vi "Trip Log and Trip Monitor.vi"(8 "error in (no error)":errorcluster, 11 "main ref":T1) -> (0 "error out":errorcluster)   [LabVIEW 2025]
uses:
  v06/controls/LAB-IQ UI Data.ctl
  Traction Loop/Traction Receipe Enum.ctl
  HEAVE vi's/Heave Write enum.ctl
  <vilib>/Utility/error.llb/Trim Whitespace One-Sided.vi
  Temperature/Temperature enum.ctl
panel:
  out "error out 4":errorcluster
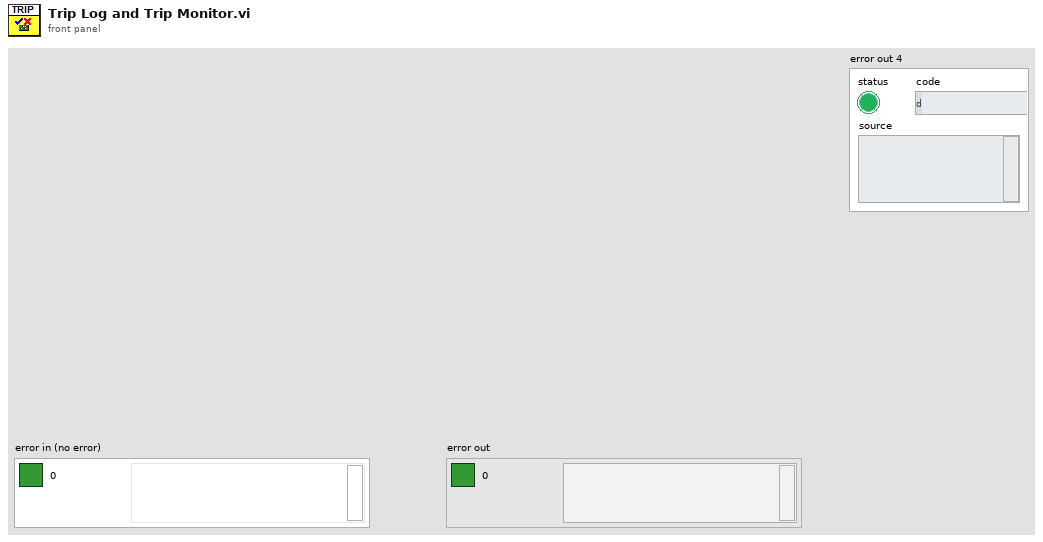
[diagram p1: front panel]
types:
  T1 = typedef "LAB-IQ UI Data.ctl" = cluster{"Main Home Screen":cluster{"GUI":refnum<vi>, "Platform Settings":refnum<vi>, "Configure":refnum<vi>, "Home":refnum<vi>, "EXIT":refnum<vi>, "service 2":refnum<vi>, "MainPage":refnum<vi>, "Analysis":refnum<vi>}, "Platform Settings":cluster{"mm/s  Surge":refnum<vi>, "Drive Error":refnum<vi>, "Disable Axis Jog Soft Limits":refnum<vi>, "mm/s  Sway":refnum<vi>, "Sway and Surge COM Status":refnum<vi>, "Heave COM Status":refnum<vi>, "Enable Platform":refnum<vi>, "Surge Forward Main":refnum<vi>, "Sway Right Main":refnum<vi>, "Sway Left Main":refnum<vi>, "Heave Down Main":refnum<vi>, "Heave Up main":refnum<vi>, "mm/s Heave":refnum<vi>, "mm/sec":refnum<vi>, "mm":refnum<vi>, "Surge Backward Main":refnum<vi>}, "Analysis Screen":cluster{"Analysis Home":refnum<vi>, "Surface Analysis":refnum<vi>, "Imaging":refnum<vi>, "Image Analysis":refnum<vi>, "Post Analysis":refnum<vi>}, "Config Screen":cluster{"Select Load Head":refnum<vi>, "Notes :":refnum<vi>, "FILE":refnum<vi>, "Sample ID :":refnum<vi>, "Operator ID :":refnum<vi>, "Operator Name :":refnum<vi>, "Auto":refnum<vi>}, "Motion Module":cluster{"zNL":refnum<vi>, "NL disp":refnum<vi>, "Rotary Tab":refnum<vi>, "Motion Direction:  3":refnum<vi>, "E.Velocity 2":refnum<vi>, "e.v/ssr 2":refnum<vi>, "Enter Fixed E.Velocity 2":refnum<vi>, "Enter Final SRR 2":refnum<vi>, "Enter initial SRR 2":refnum<vi>, "Enter Fixed SRR 2":refnum<vi>, "Enter the Final E.Velocity (m/s) 2":refnum<vi>, "Enter initial E.Velocity (m/s) 2":refnum<vi>, "Final Speed (RPM) 3":refnum<vi>, "Initial Speed (RPM) 2":refnum<vi>, "Enter the Final Velocity (m/s) 3":refnum<vi>, "Enter initial Velocity (m/s)  3":refnum<vi>, "Ramp Up 2":refnum<vi>, "TEST SELECTION":refnum<vi>, "SPEED SELECTION : ":refnum<vi>, "Angular Oscillation Set":refnum<vi>, "Traction":refnum<vi>, "Step Speed":refnum<vi>, "StepTable For Load-Speed":refnum<vi>, "StepTable For Speed":refnum<vi>, "Surge Forward MM":refnum<vi>, "Surge Backward MM":refnum<vi>, "M3 Image":refnum<vi>, "String 39":refnum<vi>, "Sway Left MM":refnum<vi>, "Sway Right MM":refnum<vi>, "Disable Axis Jog Soft Limits":refnum<vi>, "mm":refnum<vi>, "Heave Down MM":refnum<vi>, "Heave Up MM":refnum<vi>, "Wear Track Diameter (mm)":refnum<vi>, "Set WTD":refnum<vi>, "HomeScratch":refnum<vi>, "HomeRot":refnum<vi>, "PlaceModule":refnum<vi>, "Enter the Angle (Deg)":refnum<vi>, "Enter the Frequency (Hz)":refnum<vi>, "Motion Mode:":refnum<vi>, "LR Sway":refnum<vi>, "Rot Hor":refnum<vi>, "Scratch":refnum<vi>, "LR Cam":refnum<vi>, "MMBack":refnum<vi>, "MMNext":refnum<vi>, "Rot Ver":refnum<vi>, "Rotary Module Selection":refnum<vi>, "calculate rotary":refnum<vi>, "SPEED SELECTION : rotary":refnum<vi>, "Import 2":refnum<vi>, "Save 2":refnum<vi>, "File Path :  2":refnum<vi>, "String 45":refnum<vi>, "StepTable For Speed 3":refnum<vi>, "Enter the Speed(mm/sec)":refnum<vi>, "Enter the Speed(RPM)":refnum<vi>, "Enter Scratch Speed (mm/s):":refnum<vi>, "SwaySpeed Set":refnum<vi>, "Scartch Offset":refnum<vi>, "Motion type:":refnum<vi>, "HomeScratch 2":refnum<vi>, "Enter Scratch length (mm):":refnum<vi>, "Wear Track Diameter":refnum<vi>, "Rotary Speed Exced":refnum<vi>, "Scratch Mode":refnum<vi>, "No of Scratch":refnum<vi>}, "Environmental control":cluster{"Humidity  Status  3":refnum<vi>, "Low Temp  Status  2":refnum<vi>, "TK4 status 2":refnum<vi>, "Stage Temperature":refnum<vi>, "Sample Temperature":refnum<vi>, "Humidity (Amb)":refnum<vi>, "Clear List":refnum<vi>, "Add to list":refnum<vi>, "Wear":refnum<vi>, "Vibration":refnum<vi>, "Humidity (Chamber)":refnum<vi>, "Temperature (Chamber)":refnum<vi>, "ECR ":refnum<vi>, "Temperature (Amb)":refnum<vi>, "Microphone":refnum<vi>, "Acoustic Emission 3":refnum<vi>, "SNext":refnum<vi>, "APBack":refnum<vi>, "Enter the Temperature (°C):":refnum<vi>, "Enter the Stage \nTemperature (°C):":refnum<vi>, "Enter the Humidity (%Rh):":refnum<vi>, "Low Temp":refnum<vi>, "High Temp":refnum<vi>, "Humidity":refnum<vi>, "Sensors Picked":refnum<vi>}, "About Screen":cluster{"Password":refnum<vi>, "Home Service":refnum<vi>, "Advanced Setting":refnum<vi>, "About Tab":refnum<vi>, "ECR Port:":refnum<vi>, "Ramp Port:":refnum<vi>, "Installation/Replacement completed":refnum<vi>, "Loahead":refnum<vi>, "Heave and Surge COM Port:":refnum<vi>, "Sway COM Port:":refnum<vi>, "Temp Modbus:":refnum<vi>, "Humidity Port:":refnum<vi>, "Edit Gain Constants":refnum<vi>, "Save Gain Constants":refnum<vi>}, "Main Screen":cluster{"Main Screen Tab":refnum<vi>, "Angle and Frequency":refnum<vi>, "Stroke (mm)":refnum<vi>, "Angle (Deg)":refnum<vi>, "Main Speed Tab":refnum<vi>, "MTM MOTOR DISPLAY":refnum<vi>, "Disc Speed (m/sec)":refnum<vi>, "Ball Speed (m/sec)":refnum<vi>, "Disc Speed (RPM)":refnum<vi>, "Ball Speed (RPM)":refnum<vi>, "SPEED TAB":refnum<vi>, "Speed (m/sec)":refnum<vi>, "Set Speed (m/sec)":refnum<vi>, "Speed (RPM)":refnum<vi>, "Set Speed":refnum<vi>, "Time Tab":refnum<vi>, "Time ( HH:MM:SS ) 2":refnum<vi>, "Test Duration":refnum<vi>, "Test Duration 4":refnum<vi>, "TEST CYCLE":refnum<vi>, "TOTAL CYCLES":refnum<vi>, "Set Load (N)":refnum<vi>, "Temp Tabs":refnum<vi>, "Heater":refnum<vi>, "TK4 status":refnum<vi>, "ChamberTemp":refnum<vi>, "SetTmp":refnum<vi>, "Controller  Status":refnum<vi>, "ChamberTemp 2":refnum<vi>, "SetTmp 2":refnum<vi>, "Controller  Status 2":refnum<vi>, "ChamberTemp 3":refnum<vi>, "SetTmp 3":refnum<vi>, "Cooling":refnum<vi>, "Load Communication":refnum<vi>, "Ambient \nTemperature":refnum<vi>, "HumCOMStatus":refnum<vi>, "Ambient\n Humidity":refnum<vi>, "Freq (Hz)":refnum<vi>, "Load En":refnum<vi>, "NLt":refnum<vi>, "zNL 2":refnum<vi>, "Humidity On":refnum<vi>, "humidity disp":refnum<vi>, "Set Humidity":refnum<vi>, "NL disp 2":refnum<vi>, "Humidity On 2":refnum<vi>, "humidity disp 2":refnum<vi>, "Set Humidity 2":refnum<vi>, "NL disp 3":refnum<vi>, "AppLoadSeq scratch":refnum<vi>, "Stop Scratch":refnum<vi>, "ClrLog":refnum<vi>, "Trip Log":refnum<vi>, "STOP":refnum<vi>, "Start Test":refnum<vi>, "Test status":refnum<vi>, "AR Led":refnum<vi>, "Data":refnum<vi>, "Health":refnum<vi>, "Sway COM Status":refnum<vi>, "Heave COM Status":refnum<vi>, "Grp Tab":refnum<vi>, "Sub Graph":refnum<vi>, "SD (mm)":refnum<vi>, "Siliding distance Reset Graph":refnum<vi>, "SDGp":refnum<vi>, "Humidity Reset Graph":refnum<vi>, "HumrGp":refnum<vi>, "Acoustic Emission (mV)":refnum<vi>, "Aqucostic Reset Graph":refnum<vi>, "gACQUOS":refnum<vi>, "ECR RESET":refnum<vi>, "ECR":refnum<vi>, "Temperature Reset":refnum<vi>, "Acoustic Emission (mV) 2":refnum<vi>, "Aqucostic Reset Graph 2":refnum<vi>, "gACQUOS 2":refnum<vi>, "ECR RESET 2":refnum<vi>, "ECR 2":refnum<vi>, "Temperature Reset 2":refnum<vi>, "Temperature (deg c)":refnum<vi>, "Speed Reset Graph":refnum<vi>, "Speed Tab":refnum<vi>, "MTM DISC  SPEED":refnum<vi>, "MTM BALL SPEED":refnum<vi>, "speed mm/sec":refnum<vi>, "Hymidity":refnum<vi>, "Humidity Disable trip":refnum<vi>, "CoF Trip  2":refnum<vi>, "Depth Trip":refnum<vi>, "Weart Deapth":refnum<vi>, "Depth Reset Graph":refnum<vi>, "Weart":refnum<vi>, "Depthz":refnum<vi>, "Depth (µm)":refnum<vi>, "WearGp":refnum<vi>, "NL Trip 2":refnum<vi>, "Load pid":refnum<vi>, "Load Disable Trip":refnum<vi>, "Load Reset Graph":refnum<vi>, "NL Display 4":refnum<vi>, "Main Chart 3":refnum<vi>, "BACK":refnum<vi>, "Depth Trip 2":refnum<vi>, "COF TRIP ":refnum<vi>, "Friction Force (N)":refnum<vi>, "FF Reset Graph":refnum<vi>, "FF Disable Trip":refnum<vi>, "FF TRIP":refnum<vi>, "COF Disable Trip":refnum<vi>, "COF Reset Graph":refnum<vi>, "Start Test Temp":refnum<vi>, "zFF":refnum<vi>, "Friction Force (N) Graph":refnum<vi>, "Coefficient of Friction":refnum<vi>, "Scratch Start Test":refnum<vi>, "FF Tab":refnum<vi>, "Cyclic Friction Force (N)":refnum<vi>, "CZ FF":refnum<vi>, "Cyclic Friction Force (N) Graph":refnum<vi>, "Cyclic Coefficient of Friction":refnum<vi>, "Cyclic FF TRIP":refnum<vi>, "Cyclic FF Disable Trip":refnum<vi>, "cyclic COF Disable Trip":refnum<vi>, "cyclic COF TRIP":refnum<vi>, "cyclic COF Reset Graph":refnum<vi>, "Cyclic FF Reset Graph":refnum<vi>, "Test Trip":refnum<vi>, "Multi Scratch Pass":refnum<vi>, "Scratch Start Recording":refnum<vi>, "Coefficient of Friction 2":refnum<vi>, "Acoustic Emission":refnum<vi>, "Friction Force (N) 2":refnum<vi>, "Depth (Microns)":refnum<vi>, "Normal Load ( N )":refnum<vi>}, "Loading":cluster{"Indentation":refnum<vi>, "Reference Sample":refnum<vi>, "Load Cell Communication Slide":refnum<vi>, "com 3":refnum<vi>, "com":refnum<vi>, "DecaForce COM Status":refnum<vi>, "Update":refnum<vi>, "Clear 3":refnum<vi>, "seq":refnum<vi>, "Stribeck table":refnum<vi>, "Stribeck Table  For loading":refnum<vi>, "Loading Mode":refnum<vi>, "Enter the Final Load (N)":refnum<vi>, "Enter the CoF Trip":refnum<vi>, "Enter the Friction Force Trip":refnum<vi>, "Enter the Normal load Trip":refnum<vi>, "Enter the Load  (N)":refnum<vi>, "KiloForce":refnum<vi>, "DecaForce ":refnum<vi>, "MicroForce":refnum<vi>, "LHBack":refnum<vi>, "LHNext":refnum<vi>, "Enter the Loading Rate (N/min)":refnum<vi>, "Message":refnum<vi>, "Warning 2":refnum<vi>, "SSP 0.75":refnum<vi>, "SSP 0.5":refnum<vi>, "SSP 0.3":refnum<vi>, "Warning":refnum<vi>, "gui GIF":refnum<vi>, "Communication is established":refnum<vi>, "AppLoad 4":refnum<vi>, "Multipoint":refnum<vi>, "Load Selection":refnum<vi>}, "PID":cluster{"Ramp":refnum<vi>, "Vertical load (N)":refnum<vi>, "apply load":refnum<vi>, "apply load 2":refnum<vi>, "Enter ByPass Load":refnum<vi>, "Bypass Load":refnum<vi>, "gFF Rot":refnum<vi>}, "Config Parameters":cluster{"Tab Control 3":refnum<vi>, "Tab Control 19":refnum<vi>, "SAMPLES":refnum<vi>, "Re-initilaize":refnum<vi>, "Filter ON/OFF":refnum<vi>, "TracHomeSurgeOffsetCounts 10MM":refnum<vi>, "TracHomeSwayOffsetCounts 10MM":refnum<vi>, "Acoustic Emission:":refnum<vi>, "Apply Filter (FF)":refnum<vi>, "Filter% 2":refnum<vi>, "Apply Filter (Load)":refnum<vi>, "Filter% ":refnum<vi>, "Sway distance (mm)":refnum<vi>, "Surge distance (mm)":refnum<vi>, "DataSavingLoopDelay(ms)":refnum<vi>, "SAVE 2":refnum<vi>, "Enter Distance":refnum<vi>, "Sway Counts:":refnum<vi>, "Distance (mm): 3":refnum<vi>, "Surge Counts:":refnum<vi>, "Distance (mm): 2":refnum<vi>, "Distance (mm):":refnum<vi>, "Heave Counts:":refnum<vi>, "LRMHomeSurgeOffsetCounts":refnum<vi>, "LRMHomeSwayOffsetCounts":refnum<vi>, "TracHomeSurgeOffsetCounts 20MM":refnum<vi>, "TracHomeSwayOffsetCounts 20MM":refnum<vi>, "RotHomeSwayOffsetCounts":refnum<vi>, "RotHomeSurgeOffsetCounts":refnum<vi>, "Heave distance":refnum<vi>, "Zmm":refnum<vi>, "Heave Pulses/mm":refnum<vi>, "Surge Pulses/mm":refnum<vi>, "Sway Pulses/mm":refnum<vi>, "Heave Pitch":refnum<vi>, "Surge Pitch":refnum<vi>, "Sway Pitch":refnum<vi>, "Heave PPR":refnum<vi>, "Surge PPR":refnum<vi>, "Sway PPR":refnum<vi>, "Tab Control 5":refnum<vi>, "Tab Control 14":refnum<vi>, "Tab Control 26":refnum<vi>, "AE":refnum<vi>, "Heave Loop Delay":refnum<vi>, "Heave PID Speed":refnum<vi>, "Surge Jog Speed":refnum<vi>, "Heave Jog Speed":refnum<vi>, "Sway Loop Delay":refnum<vi>, "Sway PID Speed":refnum<vi>, "Sway Jog Speed":refnum<vi>, "DEPTH TRIP VALUE":refnum<vi>, "LOAD TRIP VALUE":refnum<vi>, "DEPTH TRIP   ENABLE":refnum<vi>, "LOAD TRIP  ENABLE":refnum<vi>, "CYCLIC FF TRIP VALUE":refnum<vi>, "FF TRIP VALUE":refnum<vi>, "CYCLIC CoF TRIP VALUE":refnum<vi>, "COF TRIP VALUE":refnum<vi>, "CYCLIC COF TRIP  ENABLE":refnum<vi>, "CYCLIC FF TRIP  ENABLE":refnum<vi>, "FF TRIP  ENABLE":refnum<vi>, "COF TRIP  ENABLE":refnum<vi>, "JOG TRIP LOAD VALUE (N)":refnum<vi>, "Rotary Vertical":refnum<vi>, "Traction":refnum<vi>, "Scratch":refnum<vi>, "LRM CAM":refnum<vi>, "Sway LRM":refnum<vi>, "Rotary Horizontal":refnum<vi>, "SURGE SPEED":refnum<vi>, "SURGE BACKWARD COUNT":refnum<vi>, "SURGE FORWARD COUNT":refnum<vi>, "Start Button":refnum<vi>}, "Loading Com Port":cluster{"ClearAll":refnum<vi>, "Mz(Nm)":refnum<vi>, "My(Nm)":refnum<vi>, "Mx(Nm)":refnum<vi>, "Save Dwell":refnum<vi>, "Acq Delay (ms)":refnum<vi>, "Burst Delay (ms)":refnum<vi>, "model":refnum<vi>, "SN":refnum<vi>, "FFx(N)":refnum<vi>, "Sensor IP":refnum<vi>, "Port":refnum<vi>, "FFy(N)":refnum<vi>, "Load(N)":refnum<vi>, "delete Handle":refnum<vi>, "Create Handle":refnum<vi>, "ft_data":refnum<vi>, "ft_range":refnum<vi>, "ft_data 2":refnum<vi>, "stop 6":refnum<vi>, "running_flag":refnum<vi>, "ft_udp_handle":refnum<vi>, "get-data-return":refnum<vi>, "get-range-return":refnum<vi>, "zero-return":refnum<vi>, "filter-return":refnum<vi>, "initial-return":refnum<vi>, "deleteHandle-result":refnum<vi>, "Load Cell Temp":refnum<vi>, "Load Cell":refnum<vi>, "ZeroAll":refnum<vi>, "FORCE (N)":refnum<vi>, "TORQUE (N-m)":refnum<vi>, "Load Cell Link":refnum<vi>}, "Heave AND Surge":cluster{"SURGE POSE":refnum<vi>, "error out Read":refnum<vi>, "HEAVE POSE":refnum<vi>, "State":refnum<vi>, "Homed":refnum<vi>, "Sequence ID":refnum<vi>, "error out Write":refnum<vi>, "faultCode":refnum<vi>, "Ack ID":refnum<vi>, "SPEED":refnum<vi>, "Distance":refnum<vi>, "Mode Command":refnum<vi>, "Heave and Surge Read":refnum<vi>, "Read Heave Temp":refnum<vi>, "Spare 15":refnum<vi>, "Spare 14":refnum<vi>, "Spare 13":refnum<vi>, "Spare 12":refnum<vi>, "Spare 11":refnum<vi>, "Spare 10":refnum<vi>, "Spare 9":refnum<vi>, "Spare 8":refnum<vi>, "Spare 7":refnum<vi>, "Spare 4":refnum<vi>, "Spare 3":refnum<vi>, "Spare 2":refnum<vi>, "Humidity":refnum<vi>, "Temp":refnum<vi>, "Node Id":refnum<vi>, "Spare 1":refnum<vi>, "SPARE 4":refnum<vi>, "SPARE 3":refnum<vi>, "SPARE 2":refnum<vi>, "SPARE 1":refnum<vi>, "fwMajor":refnum<vi>, "fwMinor":refnum<vi>, "Manual Write":refnum<vi>, "Heave and Surge Write":refnum<vi>, "SPARE 5":refnum<vi>, "Reserved ":refnum<vi>, "SPARE 8":refnum<vi>, "SPARE 6":refnum<vi>, "SPARE 7":refnum<vi>, "SPARE 17":refnum<vi>, "SPARE 16":refnum<vi>, "SPARE 15":refnum<vi>, "SPARE 14":refnum<vi>, "SPARE 13":refnum<vi>, "SPARE 12":refnum<vi>, "SPARE 11":refnum<vi>, "SPARE 10":refnum<vi>, "SPARE 9":refnum<vi>, "System UPTIME":refnum<vi>, "Missed Packets":refnum<vi>, "faultCode Surge Right":refnum<vi>, "faultCode Surge Left":refnum<vi>, "faultCode Heave":refnum<vi>, "UPLINK HEAVE":refnum<vi>, "DOWNLINK HEAVE":refnum<vi>}, "New PID LOGIC":cluster{"Fine Tune Zone":refnum<vi>, "PID SDelay":refnum<vi>, "Max_pos_limit":refnum<vi>, "Min_pos_limit":refnum<vi>, "i_limit":refnum<vi>, "pct_scale":refnum<vi>, "Deadband":refnum<vi>, "Kd":refnum<vi>, "Ki":refnum<vi>, "Kp":refnum<vi>, "Current Position":refnum<vi>, "Set Load":refnum<vi>, "Current Load":refnum<vi>, "Pulse delta":refnum<vi>, "Init Step":refnum<vi>, "Max Step Linit":refnum<vi>, "min_deadband_floor":refnum<vi>, "dynamic_spindle_noise_scalar":refnum<vi>, "min_finetune_floor":refnum<vi>, "filter_alpha":refnum<vi>, "PID":refnum<vi>}, "SWAY ":cluster{"fwMajor":refnum<vi>, "Homed":refnum<vi>, "Rotary POSE":refnum<vi>, "State":refnum<vi>, "SWAY POSE":refnum<vi>, "Ack ID":refnum<vi>, "faultCode":refnum<vi>, "Node Id":refnum<vi>, "fwMinor":refnum<vi>, "Spare 6":refnum<vi>, "Spare 5":refnum<vi>, "Spare 4":refnum<vi>, "Spare 3":refnum<vi>, "Spare 2":refnum<vi>, "Spare 1":refnum<vi>, "Spare 7":refnum<vi>, "SPARE  5":refnum<vi>, "error out Write  SWAY ":refnum<vi>, "error out Read SWAY ":refnum<vi>, "Manual Write SWAY ":refnum<vi>, "SWAY WRITE":refnum<vi>, "SPARE  4":refnum<vi>, "SPARE  3":refnum<vi>, "SPARE 2":refnum<vi>, "SPARE 1":refnum<vi>, "Spare 15":refnum<vi>, "Spare 14":refnum<vi>, "Spare 13":refnum<vi>, "Spare 12":refnum<vi>, "Spare 11":refnum<vi>, "Spare 9":refnum<vi>, "Spare 8":refnum<vi>, "SPEED":refnum<vi>, "Distance":refnum<vi>, "Mode Command":refnum<vi>, "Sequence ID":refnum<vi>, "SWAY READ":refnum<vi>, "Spare 10":refnum<vi>, "Read SWAY Temp":refnum<vi>, "faultCode Sway ":refnum<vi>, "Missed Packets":refnum<vi>, "System UPTIME sway":refnum<vi>, "SPARE 6":refnum<vi>, "SPARE 7":refnum<vi>, "SPARE 9":refnum<vi>, "SPARE 11":refnum<vi>, "SPARE 10":refnum<vi>, "SPARE 8":refnum<vi>, "SPARE 13":refnum<vi>, "SPARE 12":refnum<vi>, "SPARE 17":refnum<vi>, "SPARE 16":refnum<vi>, "SPARE 15":refnum<vi>, "SPARE 14":refnum<vi>, "Reserved":refnum<vi>, "faultCode Rotary":refnum<vi>, "UPLINK SWAY":refnum<vi>, "DOWNLINK SWAY":refnum<vi>}, "Analysis Screen":cluster{"Analysis Home":refnum<vi>, "Refresh 2":refnum<vi>, "MEAN 4":refnum<vi>, "SD 4":refnum<vi>, "VARIANCE 4":refnum<vi>, "MEAN  3":refnum<vi>, "SD  3":refnum<vi>, "VARIANCE  3":refnum<vi>, "MEAN 2":refnum<vi>, "SD  2":refnum<vi>, "VARIANCE 2":refnum<vi>, "MEAN":refnum<vi>, "SD":refnum<vi>, "VARIANCE":refnum<vi>, "File 4 Discription":refnum<vi>, "OPEN 4":refnum<vi>, "File Name 4":refnum<vi>, "OPEN 3":refnum<vi>, "File 3 Discription":refnum<vi>, "File Name 3":refnum<vi>, "Y-AXIS":refnum<vi>, "X-AXIS":refnum<vi>, "XY Graph":refnum<vi>, "File Name 2":refnum<vi>, "File Name 1":refnum<vi>, "OPEN 2":refnum<vi>, "OPEN 1":refnum<vi>, "File 1 Discription ":refnum<vi>, "File 2 Discription":refnum<vi>, "Export":refnum<vi>, "File Format":refnum<vi>}, "Traction":cluster{"faultCode Traction 2":refnum<vi>, "faultCode Traction 1":refnum<vi>, "Missed Packets":refnum<vi>, "System UPTIME Traction":refnum<vi>, "SPARE 17":refnum<vi>, "SPARE 16":refnum<vi>, "SPARE 15":refnum<vi>, "SPARE 14":refnum<vi>, "SPARE 13":refnum<vi>, "SPARE 12":refnum<vi>, "SPARE 11":refnum<vi>, "SPARE 10":refnum<vi>, "SPARE 9":refnum<vi>, "SPARE 8":refnum<vi>, "SPARE 7":refnum<vi>, "SPARE 6":refnum<vi>, "Reserved":refnum<vi>, "SPARE  5":refnum<vi>, "Manual Write TRACTION":refnum<vi>, "TRACTION WRITE":refnum<vi>, "SPARE  4":refnum<vi>, "SPARE  3":refnum<vi>, "SPARE 2":refnum<vi>, "SPARE 1":refnum<vi>, "Spare 7":refnum<vi>, "Spare 6":refnum<vi>, "Spare 5":refnum<vi>, "Spare 4":refnum<vi>, "Spare 2":refnum<vi>, "Spare 1":refnum<vi>, "Node Id":refnum<vi>, "Read TRACTION Temp":refnum<vi>, "fwMinor":refnum<vi>, "fwMajor":refnum<vi>, "faultCode":refnum<vi>, "TRACTION POSE":refnum<vi>, "TRACTION POSE 2":refnum<vi>, "Homed":refnum<vi>, "State":refnum<vi>, "Ack ID":refnum<vi>, "SPEED":refnum<vi>, "Distance":refnum<vi>, "Mode Command":refnum<vi>, "Sequence ID":refnum<vi>, "error out Read TRACTION":refnum<vi>, "error out Write  TRACTION":refnum<vi>, "TRACTION READ":refnum<vi>, "Spare 3":refnum<vi>, "Downlink traction":refnum<vi>, "Uplink Traction":refnum<vi>}, "Traction reciepe":cluster{"SRR Sweep Range (%) Stribeck":refnum<vi>, "Traction Receipe":refnum<vi>, "Total Execution Time":refnum<vi>, "Total Steps":refnum<vi>, "Duration / Step (s)  Stribeck":refnum<vi>, "STRIBECK Fixed SRR List (%)":refnum<vi>, "Duration / Step (s) Traction":refnum<vi>, "SRR Sweep Range (%) traction":refnum<vi>, "Rolling Speed (mm/s)":refnum<vi>, "Temperature Stages (°C)":refnum<vi>, "Ball Load (N)":refnum<vi>, "Lubricant Name":refnum<vi>, "Profile File Name":refnum<vi>, "SET entrainment Velocity":refnum<vi>, "Test Array Size":refnum<vi>, "SRR INDEX [ STRIBECK]":refnum<vi>, "Stribeck Size":refnum<vi>, "SET SRR":refnum<vi>, "ELAPSED TIMER ":refnum<vi>, "BALL SET RPM":refnum<vi>, "DISC SET RPM":refnum<vi>, "SET LOAD":refnum<vi>, "TEMPERATURE READ":refnum<vi>, "SET TEMPERATURE":refnum<vi>, "Traction Size":refnum<vi>, "DISC SPEED (rpm)":refnum<vi>, "BALL SPEED (rpm)":refnum<vi>, "BALL WEAR TRACK":refnum<vi>, "DISC WEARTRACK":refnum<vi>, "SRR INDEX [ TRACTION]":refnum<vi>, "Start Index Type":refnum<vi>, "Enum - Menu":refnum<vi>, "Ball (mm/sec)":refnum<vi>, "Disc (mm/sec)":refnum<vi>, "Traction Receipe Update Details":refnum<vi>}, "Traction Control":cluster{"HomeTraction":refnum<vi>, "Demo Mode Display":refnum<vi>, "Traction Message":refnum<vi>, "Traction Step Update Details":refnum<vi>, "Main Tab sequence for selection":refnum<vi>, "Ramp Tab":refnum<vi>, "e.v/ssr":refnum<vi>, "Enter Fixed E.Velocity":refnum<vi>, "Enter Final SRR":refnum<vi>, "Enter initial SRR":refnum<vi>, "Enter Fixed SRR":refnum<vi>, "Enter the Final E.Velocity (m/s)":refnum<vi>, "Enter initial E.Velocity (m/s)":refnum<vi>, "Ball WTD":refnum<vi>, "E.Velocity":refnum<vi>, "Enter the Final Velocity (m/s)":refnum<vi>, "Enter initial Velocity (m/s)":refnum<vi>, "Ramp Up   Disc":refnum<vi>, "Initial DiscSpeed (RPM)":refnum<vi>, "Final Speed (RPM) Ball":refnum<vi>, "Final Speed (RPM)":refnum<vi>, "Initial Speed (RPM) Ball":refnum<vi>, "Enter the Final Velocity (m/s) Ball":refnum<vi>, "Enter initial Velocity (m/s) Ball":refnum<vi>, "Ramp Up":refnum<vi>, "ExceedBallSpeed step":refnum<vi>, "ExceedDiscSpeed":refnum<vi>, "BallSpeed Exceed Indication":refnum<vi>, "Apply":refnum<vi>, "SPEED SELECTION : MTM":refnum<vi>, "SPEED SELECTION : MTM 2":refnum<vi>, "TEST SELECTION (MTM)":refnum<vi>, "MTM Test Selection":refnum<vi>, "File Path Tab":refnum<vi>, "File Path String":refnum<vi>, "Save":refnum<vi>, "Save  2":refnum<vi>, "Import ":refnum<vi>, "File Path :":refnum<vi>, "Step Sequence Indication Tab":refnum<vi>, "Step Sequence Indication":refnum<vi>, "Calculate Step":refnum<vi>, "StepTable":refnum<vi>, "ExceedDiscSpeed  Cinstant Speed":refnum<vi>, "ExceedBallSpeed Constant":refnum<vi>, "TEST SELECTION (MTM) 2":refnum<vi>, "SPEED SELECTION : MTM 3":refnum<vi>, "MTM Test Selection 2":refnum<vi>, "Enter the Speed (m/sec): ":refnum<vi>, "Enter the Speed (m/sec):  2":refnum<vi>, "Enter the Speed (RPM):":refnum<vi>, "Lower Spped ":refnum<vi>, "Upper":refnum<vi>, "Enter the Speed (RPM):Ball":refnum<vi>, "Disc Motion Direction: ":refnum<vi>, "Ball Motion Direction :":refnum<vi>, "Motion Mode: ":refnum<vi>, "Wear Track Diameter (mm) ":refnum<vi>, "Disc Speed Indicator":refnum<vi>, "ExceedBallSpeed":refnum<vi>}, "Acquostic":cluster{"Last Config Rejected ":refnum<vi>, "rx command count":refnum<vi>, "Current Filter Id":refnum<vi>, "Isolated Gain":refnum<vi>, "DAQ Status":refnum<vi>, "error out":refnum<vi>, "error in (no error)":refnum<vi>, "Uplink Packet":refnum<vi>, "data out":refnum<vi>, "Downlink Packet":refnum<vi>, "Gains":refnum<vi>, "Manual Write Acquostic":refnum<vi>, "Acoustic Graphs":refnum<vi>}, "ABOUT":cluster{"version":refnum<vi>, "Operating System":refnum<vi>, "Version":refnum<vi>, "Workorder":refnum<vi>, "Runtime":refnum<vi>, "Instrument Serial":refnum<vi>, "Firmware Version":refnum<vi>, "Info":refnum<vi>}, "Temperature Port":cluster{"Temperature":refnum<vi>, "error out Temperature":refnum<vi>, "READ TEMPERATURE":refnum<vi>}}
  T2 = typedef "Temperature enum.ctl" = enum16{"Init", "read", "write", "close", "error_init"}
  T3 = cluster{"Sequence ID":u16, "Mode Command":u8, "Distance":sgl, "SPEED":sgl, "Reserved":sgl, "SPARE 1":u8, "SPARE 2":u8, "SPARE 3":u8, "SPARE 4":u8, "SPARE 5":u8, "SPARE 6":u8, "SPARE 7":u8, "SPARE 8":u8, "SPARE 9":u8, "SPARE 10":u8, "SPARE 11":u8, "SPARE 12":u8, "SPARE 13":u8, "SPARE 14":u8, "SPARE 15":u8, "SPARE 16":u8, "SPARE 17":u8}
  T4 = typedef "Heave Write enum.ctl" = enum16{"INIT", "WRITE", "CLOSE", "REINIT"}
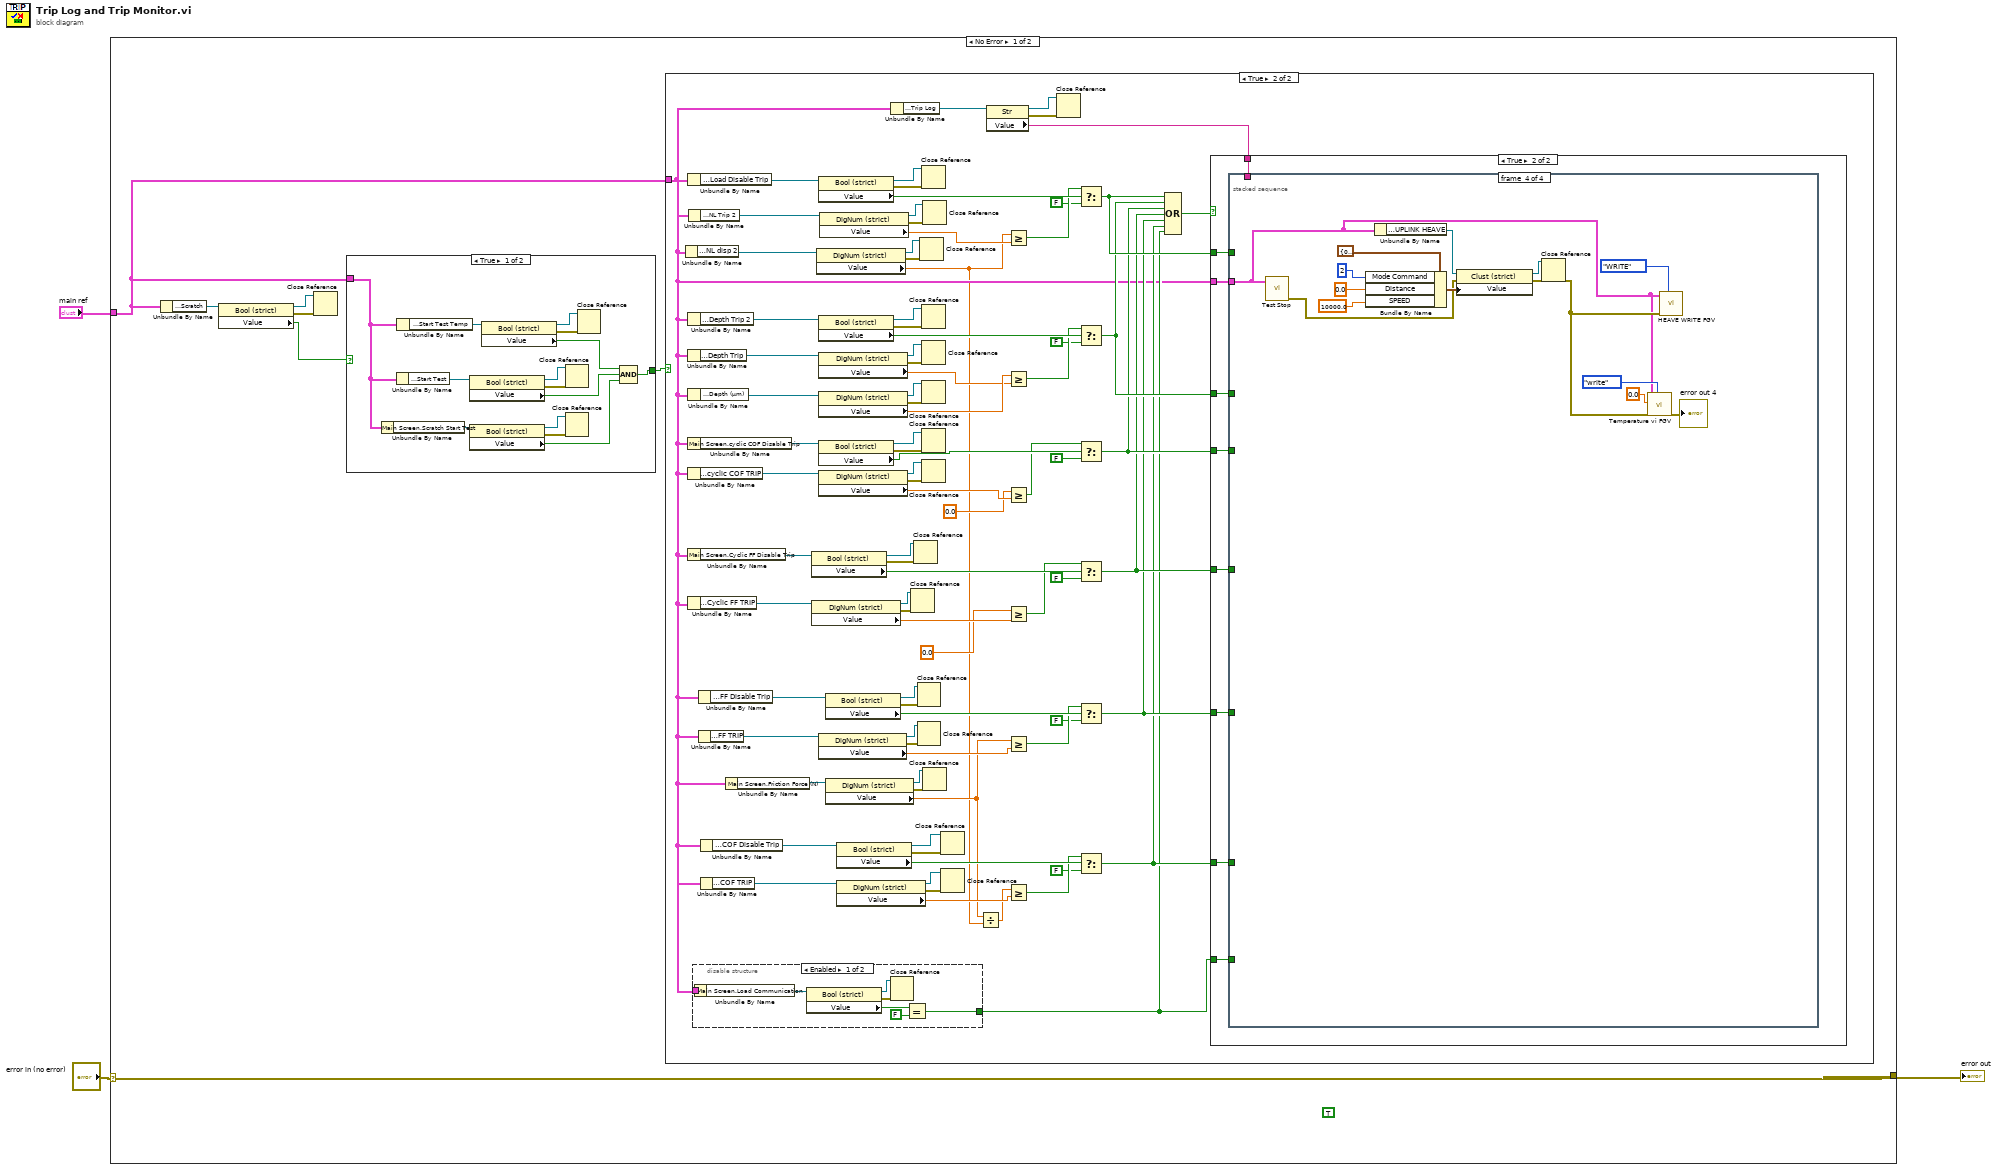
[diagram p0: block diagram]
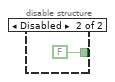
[diagram p3: hidden frame]
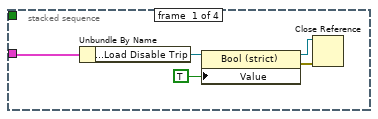
[diagram p5: hidden frame]
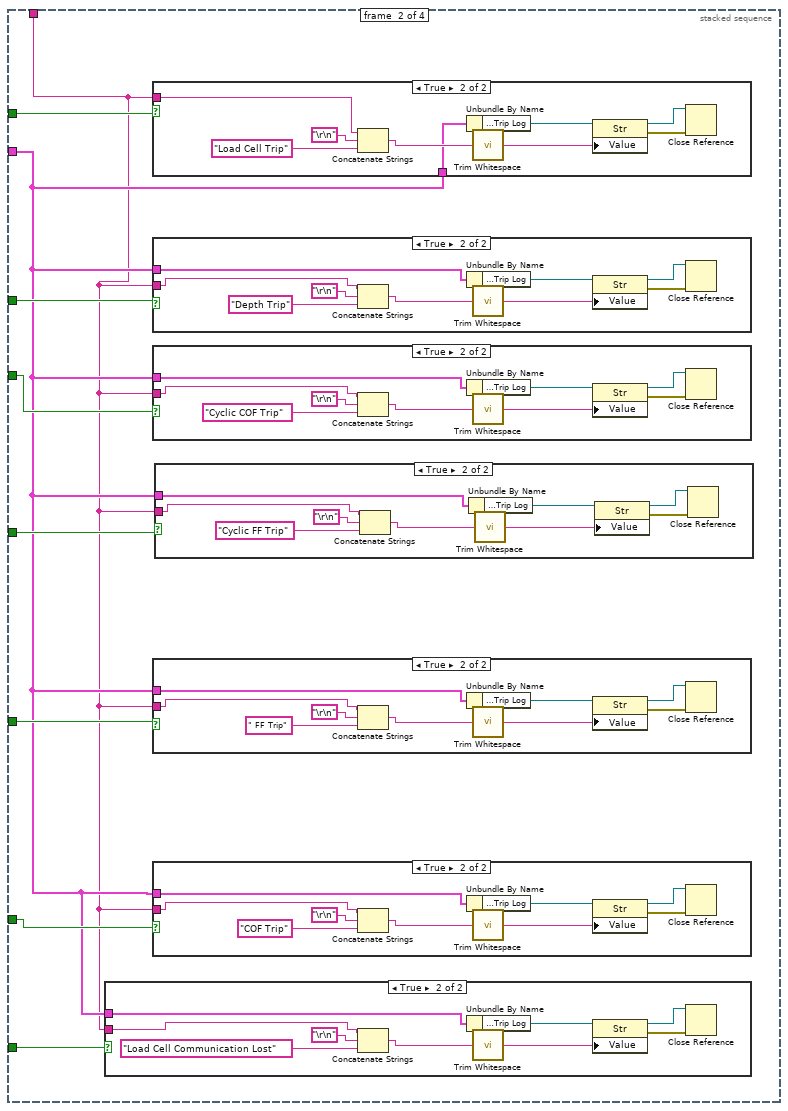
[diagram p6: hidden frame]
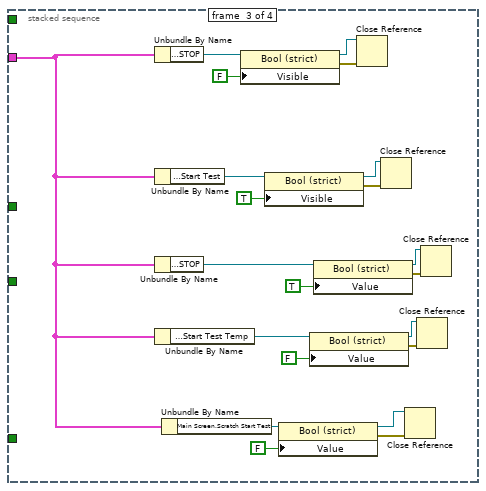
[diagram p14: hidden frame]
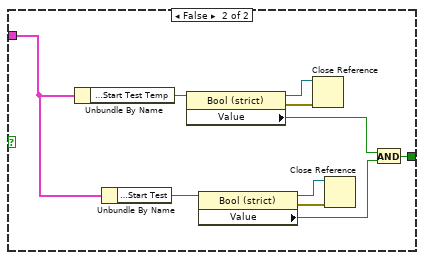
[diagram p15: hidden frame]
diagram:
  n1 = case shown="No Error" "error in (no error)" {
    selector: "error in (no error)" -> [w10 _]
    tunnel: [w10 _] -> w2
    tunnel: "main ref" -> [w9 _]
    frame No Error {
      (unwired) TRUE
      n2 = Unbundle By Name(w9) -> ("Motion Module.Scratch"=w7:refnum<vi>)
      n3 = property class="Bool (strict)"(reference=w7) -> (reference out=w8:refnum<vi>, error out=w6:errorcluster, "Value"=w5:bool)  [unwired: 1 in]
      n4 = Close Reference(reference=w8, error in (no error)=w6) -> ()  [unwired: 1 out]
      n5 = case shown="True" w5 {
        tunnel: w9 -> [w230 w246]
        tunnel: [w234 w244] -> w4
        frame True {
          n6 = Unbundle By Name(w230) -> ("Main Screen.Scratch Start Test"=w232:refnum<vi>)
          n7 = Unbundle By Name(w230) -> ("Main Screen.Start Test"=w238:refnum<vi>)
          n8 = Unbundle By Name(w230) -> ("Main Screen.Start Test Temp"=w241:refnum<vi>)
          n9 = property class="Bool (strict)"(reference=w238) -> (reference out=w237:refnum<vi>, error out=w239:errorcluster, "Value"=w235:bool)  [unwired: 1 in]
          n10 = property class="Bool (strict)"(reference=w232) -> (reference out=w233:refnum<vi>, error out=w231:errorcluster, "Value"=w229:bool)  [unwired: 1 in]
          n11 = property class="Bool (strict)"(reference=w241) -> (reference out=w242:refnum<vi>, error out=w240:errorcluster, "Value"=w236:bool)  [unwired: 1 in]
          n12 = Close Reference(reference=w237, error in (no error)=w239) -> ()  [unwired: 1 out]
          n13 = Close Reference(reference=w233, error in (no error)=w231) -> ()  [unwired: 1 out]
          n14 = Close Reference(reference=w242, error in (no error)=w240) -> ()  [unwired: 1 out]
          n15 = Compound Arithmetic op=AND(w236, w235, w229) -> (w234:bool)
        }
        frame False {
          n16 = Unbundle By Name(w246) -> ("Main Screen.Start Test Temp"=w251:refnum<vi>)
          n17 = Unbundle By Name(w246) -> ("Main Screen.Start Test"=w248:refnum<vi>)
          n18 = property class="Bool (strict)"(reference=w251) -> (reference out=w252:refnum<vi>, error out=w250:errorcluster, "Value"=w245:bool)  [unwired: 1 in]
          n19 = property class="Bool (strict)"(reference=w248) -> (reference out=w247:refnum<vi>, error out=w249:errorcluster, "Value"=w243:bool)  [unwired: 1 in]
          n20 = Close Reference(reference=w252, error in (no error)=w250) -> ()  [unwired: 1 out]
          n21 = Close Reference(reference=w247, error in (no error)=w249) -> ()  [unwired: 1 out]
          n22 = And(x=w245, y=w243) -> (x .and. y?=w244:bool)
        }
      }
      n23 = case shown="True" w4 {
        tunnel: w9 -> [_ w14]
        frame False {
        }
        frame True {
          n24 = Unbundle By Name(w14) -> ("Main Screen.NL disp 2"=w98:refnum<vi>)
          n25 = Unbundle By Name(w14) -> ("Main Screen.Load Disable Trip"=w84:refnum<vi>)
          n26 = Unbundle By Name(w14) -> ("Main Screen.Depth Trip 2"=w79:refnum<vi>)
          n27 = Unbundle By Name(w14) -> ("Main Screen.Depth Trip"=w82:refnum<vi>)
          n28 = Unbundle By Name(w14) -> ("Main Screen.Depth (µm)"=w95:refnum<vi>)
          n29 = Unbundle By Name(w14) -> ("Main Screen.cyclic COF Disable Trip"=w76:refnum<vi>)
          n30 = Unbundle By Name(w14) -> ("Main Screen.cyclic COF TRIP"=w73:refnum<vi>)
          n31 = Unbundle By Name(w14) -> ("Main Screen.Cyclic FF Disable Trip"=w67:refnum<vi>)
          n32 = Unbundle By Name(w14) -> ("Main Screen.Cyclic FF TRIP"=w70:refnum<vi>)
          n33 = Unbundle By Name(w14) -> ("Main Screen.NL Trip 2"=w87:refnum<vi>)
          n34 = disable-structure shown="Enabled" {
            disable-tunnel: w14 -> [w102 _]
            disable-tunnel: [w99 FALSE] -> w20
            frame Enabled {
              n35 = Unbundle By Name(w102) -> ("Main Screen.Load Communication"=w105:refnum<vi>)
              n36 = property class="Bool (strict)"(reference=w105) -> (reference out=w103:refnum<vi>, error out=w104:errorcluster, "Value"=w101:bool)  [unwired: 1 in]
              n37 = Close Reference(reference=w103, error in (no error)=w104) -> ()  [unwired: 1 out]
              n38 = Equal?(x=w101, y=FALSE) -> (x = y?=w99:bool)
            }
            frame Disabled {
            }
          }
          n39 = Unbundle By Name(w14) -> ("Main Screen.FF Disable Trip"=w91:refnum<vi>)
          n40 = Unbundle By Name(w14) -> ("Main Screen.FF TRIP"=w65:refnum<vi>)
          n41 = Unbundle By Name(w14) -> ("Main Screen.COF TRIP"=w59:refnum<vi>)
          n42 = Unbundle By Name(w14) -> ("Main Screen.COF Disable Trip"=w60:refnum<vi>)
          n43 = Unbundle By Name(w14) -> ("Main Screen.Friction Force (N)"=w16:refnum<vi>)
          n44 = property class="Bool (strict)"(reference=w67) -> (reference out=w68:refnum<vi>, error out=w66:errorcluster, "Value"=w53:bool)  [unwired: 1 in]
          n45 = property class="DigNum (strict)"(reference=w70) -> (reference out=w69:refnum<vi>, error out=w71:errorcluster, "Value"=w43:dbl)  [unwired: 1 in]
          n46 = property class="DigNum (strict)"(reference=w98) -> (reference out=w90:refnum<vi>, error out=w97:errorcluster, "Value"=w11:dbl)  [unwired: 1 in]
          n47 = property class="DigNum (strict)"(reference=w65) -> (reference out=w64:refnum<vi>, error out=w63:errorcluster, "Value"=w41:dbl)  [unwired: 1 in]
          n48 = property class="Bool (strict)"(reference=w84) -> (reference out=w86:refnum<vi>, error out=w85:errorcluster, "Value"=w56:bool)  [unwired: 1 in]
          n49 = property class="Bool (strict)"(reference=w79) -> (reference out=w80:refnum<vi>, error out=w78:errorcluster, "Value"=w55:bool)  [unwired: 1 in]
          n50 = property class="DigNum (strict)"(reference=w82) -> (reference out=w81:refnum<vi>, error out=w83:errorcluster, "Value"=w47:dbl)  [unwired: 1 in]
          n51 = property class="DigNum (strict)"(reference=w95) -> (reference out=w96:refnum<vi>, error out=w94:errorcluster, "Value"=w48:dbl)  [unwired: 1 in]
          n52 = property class="Bool (strict)"(reference=w76) -> (reference out=w77:refnum<vi>, error out=w75:errorcluster, "Value"=w54:bool)  [unwired: 1 in]
          n53 = property class="DigNum (strict)"(reference=w73) -> (reference out=w72:refnum<vi>, error out=w74:errorcluster, "Value"=w45:dbl)  [unwired: 1 in]
          n54 = property class="DigNum (strict)"(reference=w87) -> (reference out=w89:refnum<vi>, error out=w88:errorcluster, "Value"=w50:dbl)  [unwired: 1 in]
          n55 = property class="Bool (strict)"(reference=w91) -> (reference out=w92:refnum<vi>, error out=w93:errorcluster, "Value"=w52:bool)  [unwired: 1 in]
          n56 = property class="DigNum (strict)"(reference=w16) -> (reference out=w17:refnum<vi>, error out=w15:errorcluster, "Value"=w12:dbl)  [unwired: 1 in]
          n57 = property class="Bool (strict)"(reference=w60) -> (reference out=w62:refnum<vi>, error out=w61:errorcluster, "Value"=w51:bool)  [unwired: 1 in]
          n58 = property class="DigNum (strict)"(reference=w59) -> (reference out=w57:refnum<vi>, error out=w58:errorcluster, "Value"=w39:dbl)  [unwired: 1 in]
          n59 = Unbundle By Name(w14) -> ("Main Screen.Trip Log"=w22:refnum<vi>)
          n60 = Close Reference(reference=w69, error in (no error)=w71) -> ()  [unwired: 1 out]
          n61 = Close Reference(reference=w68, error in (no error)=w66) -> ()  [unwired: 1 out]
          n62 = Close Reference(reference=w92, error in (no error)=w93) -> ()  [unwired: 1 out]
          n63 = Close Reference(reference=w64, error in (no error)=w63) -> ()  [unwired: 1 out]
          n64 = Close Reference(reference=w90, error in (no error)=w97) -> ()  [unwired: 1 out]
          n65 = Close Reference(reference=w86, error in (no error)=w85) -> ()  [unwired: 1 out]
          n66 = Close Reference(reference=w80, error in (no error)=w78) -> ()  [unwired: 1 out]
          n67 = Close Reference(reference=w81, error in (no error)=w83) -> ()  [unwired: 1 out]
          n68 = Close Reference(reference=w96, error in (no error)=w94) -> ()  [unwired: 1 out]
          n69 = Close Reference(reference=w77, error in (no error)=w75) -> ()  [unwired: 1 out]
          n70 = Close Reference(reference=w72, error in (no error)=w74) -> ()  [unwired: 1 out]
          n71 = Close Reference(reference=w89, error in (no error)=w88) -> ()  [unwired: 1 out]
          n72 = Close Reference(reference=w17, error in (no error)=w15) -> ()  [unwired: 1 out]
          n73 = Close Reference(reference=w62, error in (no error)=w61) -> ()  [unwired: 1 out]
          n74 = Close Reference(reference=w57, error in (no error)=w58) -> ()  [unwired: 1 out]
          n75 = Divide(x=w12, y=w11) -> (x/y=w13:dbl)
          n76 = property class="Str"(reference=w22) -> (reference out=w23:refnum<vi>, error out=w24:errorcluster, "Value"=w21:string)  [unwired: 1 in]
          n77 = Greater Or Equal?(x=w11, y=w50) -> (x >= y?=w49:bool)
          n78 = Greater Or Equal?(x=w48, y=w47) -> (x >= y?=w46:bool)
          n79 = Greater Or Equal?(x=0.0, y=w45) -> (x >= y?=w44:bool)
          n80 = Greater Or Equal?(x=0.0, y=w43) -> (x >= y?=w42:bool)
          n81 = Greater Or Equal?(x=w12, y=w41) -> (x >= y?=w40:bool)
          n82 = Greater Or Equal?(x=w13, y=w39) -> (x >= y?=w38:bool)
          n83 = Close Reference(reference=w23, error in (no error)=w24) -> ()  [unwired: 1 out]
          n84 = Select(t=w49, s=w56, f=FALSE) -> (s? t:f=w30:bool)
          n85 = Select(t=w46, s=w55, f=FALSE) -> (s? t:f=w29:bool)
          n86 = Select(t=w44, s=w54, f=FALSE) -> (s? t:f=w28:bool)
          n87 = Select(t=w42, s=w53, f=FALSE) -> (s? t:f=w27:bool)
          n88 = Select(t=w40, s=w52, f=FALSE) -> (s? t:f=w26:bool)
          n89 = Select(t=w38, s=w51, f=FALSE) -> (s? t:f=w25:bool)
          n90 = Compound Arithmetic op=OR(w30, w29, w28, w27, w26, w25, w20) -> (w31:bool)
          n91 = case shown="True" w31 {
            tunnel: w14 -> [_ w115]
            tunnel: w30 -> [_ w114]
            tunnel: w29 -> [_ w113]
            tunnel: w28 -> [_ w112]
            tunnel: w27 -> [_ w111]
            tunnel: w26 -> [_ w110]
            tunnel: w25 -> [_ w109]
            tunnel: w21 -> [_ w108]
            tunnel: w20 -> [_ w107]
            frame False {
            }
            frame True {
              n92 = stacked-sequence {
                tunnel: w115 -> [w117 w123 w193 w214]
                tunnel: w114 -> [_ w129 _ _]
                tunnel: w113 -> [_ w128 _ _]
                tunnel: w112 -> [_ w127 _ _]
                tunnel: w111 -> [_ w126 _ _]
                tunnel: w110 -> [_ w125 _ _]
                tunnel: w109 -> [_ w124 _ _]
                tunnel: w108 -> [_ w121 _ _]
                tunnel: w107 -> [_ w122 _ _]
                frame #0 {
                  n93 = Unbundle By Name(w117) -> ("Main Screen.Load Disable Trip"=w118:refnum<vi>)
                  n94 = property class="Bool (strict)"(reference=w118, "Value"=TRUE) -> (reference out=w120:refnum<vi>, error out=w119:errorcluster)  [unwired: 1 in]
                  n95 = Close Reference(reference=w120, error in (no error)=w119) -> ()  [unwired: 1 out]
                }
                frame #1 {
                  n96 = case shown="True" w122 {
                    tunnel: w123 -> [_ w131]
                    tunnel: w121 -> [_ w130]
                    frame False {
                    }
                    frame True {
                      n97 = Concatenate Strings(w130, "\r\n", "Load Cell Communication Lost" ("string")) -> (w134:string)
                      n98 = Unbundle By Name(w131) -> ("Main Screen.Trip Log"=w132:refnum<vi>)
                      n99 = call <vilib>:"Trim Whitespace.vi"("string"=w134) -> ("trimmed string"=w133:string)  [unwired: 1 in]
                      n100 = property class="Str"(reference=w132, "Value"=w133) -> (reference out=w135:refnum<vi>, error out=w136:errorcluster)  [unwired: 1 in]
                      n101 = Close Reference(reference=w135, error in (no error)=w136) -> ()  [unwired: 1 out]
                    }
                  }
                  n102 = case shown="True" w129 {
                    tunnel: w123 -> [_ w186]
                    tunnel: w121 -> [_ w184]
                    frame False {
                    }
                    frame True {
                      n103 = Concatenate Strings(w184, "\r\n", "Load Cell Trip" ("string")) -> (w188:string)
                      n104 = Unbundle By Name(w186) -> ("Main Screen.Trip Log"=w185:refnum<vi>)
                      n105 = call <vilib>:"Trim Whitespace.vi"("string"=w188) -> ("trimmed string"=w187:string)  [unwired: 1 in]
                      n106 = property class="Str"(reference=w185, "Value"=w187) -> (reference out=w189:refnum<vi>, error out=w190:errorcluster)  [unwired: 1 in]
                      n107 = Close Reference(reference=w189, error in (no error)=w190) -> ()  [unwired: 1 out]
                    }
                  }
                  n108 = case shown="True" w128 {
                    tunnel: w123 -> [_ w176]
                    tunnel: w121 -> [_ w175]
                    frame False {
                    }
                    frame True {
                      n109 = Concatenate Strings(w175, "\r\n", "Depth Trip" ("string")) -> (w179:string)
                      n110 = Unbundle By Name(w176) -> ("Main Screen.Trip Log"=w177:refnum<vi>)
                      n111 = call <vilib>:"Trim Whitespace.vi"("string"=w179) -> ("trimmed string"=w178:string)  [unwired: 1 in]
                      n112 = property class="Str"(reference=w177, "Value"=w178) -> (reference out=w180:refnum<vi>, error out=w181:errorcluster)  [unwired: 1 in]
                      n113 = Close Reference(reference=w180, error in (no error)=w181) -> ()  [unwired: 1 out]
                    }
                  }
                  n114 = case shown="True" w127 {
                    tunnel: w123 -> [_ w167]
                    tunnel: w121 -> [_ w166]
                    frame False {
                    }
                    frame True {
                      n115 = Concatenate Strings(w166, "\r\n", "Cyclic COF Trip" ("string")) -> (w170:string)
                      n116 = Unbundle By Name(w167) -> ("Main Screen.Trip Log"=w168:refnum<vi>)
                      n117 = call <vilib>:"Trim Whitespace.vi"("string"=w170) -> ("trimmed string"=w169:string)  [unwired: 1 in]
                      n118 = property class="Str"(reference=w168, "Value"=w169) -> (reference out=w171:refnum<vi>, error out=w172:errorcluster)  [unwired: 1 in]
                      n119 = Close Reference(reference=w171, error in (no error)=w172) -> ()  [unwired: 1 out]
                    }
                  }
                  n120 = case shown="True" w125 {
                    tunnel: w123 -> [_ w149]
                    tunnel: w121 -> [_ w148]
                    frame False {
                    }
                    frame True {
                      n121 = Concatenate Strings(w148, "\r\n", " FF Trip" ("string")) -> (w152:string)
                      n122 = Unbundle By Name(w149) -> ("Main Screen.Trip Log"=w150:refnum<vi>)
                      n123 = call <vilib>:"Trim Whitespace.vi"("string"=w152) -> ("trimmed string"=w151:string)  [unwired: 1 in]
                      n124 = property class="Str"(reference=w150, "Value"=w151) -> (reference out=w153:refnum<vi>, error out=w154:errorcluster)  [unwired: 1 in]
                      n125 = Close Reference(reference=w153, error in (no error)=w154) -> ()  [unwired: 1 out]
                    }
                  }
                  n126 = case shown="True" w124 {
                    tunnel: w123 -> [_ w140]
                    tunnel: w121 -> [_ w139]
                    frame False {
                    }
                    frame True {
                      n127 = Concatenate Strings(w139, "\r\n", "COF Trip" ("string")) -> (w143:string)
                      n128 = Unbundle By Name(w140) -> ("Main Screen.Trip Log"=w141:refnum<vi>)
                      n129 = call <vilib>:"Trim Whitespace.vi"("string"=w143) -> ("trimmed string"=w142:string)  [unwired: 1 in]
                      n130 = property class="Str"(reference=w141, "Value"=w142) -> (reference out=w144:refnum<vi>, error out=w145:errorcluster)  [unwired: 1 in]
                      n131 = Close Reference(reference=w144, error in (no error)=w145) -> ()  [unwired: 1 out]
                    }
                  }
                  n132 = case shown="True" w126 {
                    tunnel: w123 -> [_ w158]
                    tunnel: w121 -> [_ w157]
                    frame False {
                    }
                    frame True {
                      n133 = Concatenate Strings(w157, "\r\n", "Cyclic FF Trip" ("string")) -> (w161:string)
                      n134 = Unbundle By Name(w158) -> ("Main Screen.Trip Log"=w159:refnum<vi>)
                      n135 = call <vilib>:"Trim Whitespace.vi"("string"=w161) -> ("trimmed string"=w160:string)  [unwired: 1 in]
                      n136 = property class="Str"(reference=w159, "Value"=w160) -> (reference out=w162:refnum<vi>, error out=w163:errorcluster)  [unwired: 1 in]
                      n137 = Close Reference(reference=w162, error in (no error)=w163) -> ()  [unwired: 1 out]
                    }
                  }
                }
                frame #2 {
                  n138 = Unbundle By Name(w193) -> ("Main Screen.STOP"=w208:refnum<vi>)
                  n139 = Unbundle By Name(w193) -> ("Main Screen.Start Test"=w211:refnum<vi>)
                  n140 = Unbundle By Name(w193) -> ("Main Screen.STOP"=w202:refnum<vi>)
                  n141 = Unbundle By Name(w193) -> ("Main Screen.Start Test Temp"=w201:refnum<vi>)
                  n142 = Unbundle By Name(w193) -> ("Main Screen.Scratch Start Test"=w196:refnum<vi>)
                  n143 = property class="Bool (strict)"(reference=w208, "Visible"=FALSE) -> (reference out=w198:refnum<vi>, error out=w207:errorcluster)  [unwired: 1 in]
                  n144 = property class="Bool (strict)"(reference=w211, "Visible"=TRUE) -> (reference out=w213:refnum<vi>, error out=w212:errorcluster)  [unwired: 1 in]
                  n145 = property class="Bool (strict)"(reference=w196, "Value"=FALSE) -> (reference out=w197:refnum<vi>, error out=w195:errorcluster)  [unwired: 1 in]
                  n146 = property class="Bool (strict)"(reference=w201, "Value"=FALSE) -> (reference out=w199:refnum<vi>, error out=w200:errorcluster)  [unwired: 1 in]
                  n147 = property class="Bool (strict)"(reference=w202, "Value"=TRUE) -> (reference out=w204:refnum<vi>, error out=w203:errorcluster)  [unwired: 1 in]
                  n148 = Close Reference(reference=w198, error in (no error)=w207) -> ()  [unwired: 1 out]
                  n149 = Close Reference(reference=w213, error in (no error)=w212) -> ()  [unwired: 1 out]
                  n150 = Close Reference(reference=w197, error in (no error)=w195) -> ()  [unwired: 1 out]
                  n151 = Close Reference(reference=w199, error in (no error)=w200) -> ()  [unwired: 1 out]
                  n152 = Close Reference(reference=w204, error in (no error)=w203) -> ()  [unwired: 1 out]
                }
                frame #3 {
                  n153 = call "Test Stop.vi"("Data Cluster"=w214) -> ("error out"=w219:errorcluster)  [unwired: 10 in]
                  n154 = Bundle By Name(cluster=T3 {"Sequence ID"=0, "Mode Command"=0, "Distance"=0.0, "SPEED"=0.0, "Reserved"=0.0, "SPARE 1"=0, "SPARE 2"=0, "SPARE 3"=0, "SPARE 4"=0, "SPARE 5"=0, "SPARE 6"=0, "SPARE 7"=0, "SPARE 8"=0, "SPARE 9"=0, "SPARE 10"=0, "SPARE 11"=0, "SPARE 12"=0, "SPARE 13"=0, "SPARE 14"=0, "SPARE 15"=0, "SPARE 16"=0, "SPARE 17"=0} ("Value"), "Mode Command"=u8 2, "Distance"=sgl 0.0, "SPEED"=sgl 10000.0) -> (w227:T3)
                  n155 = Unbundle By Name(w214) -> ("Heave AND Surge.UPLINK HEAVE"=w220:refnum<vi>)
                  n156 = property on="Property Node" class="Clust (strict)"(reference=w220, error in=w219, "Value"=w227) -> (reference out=w226:refnum<vi>, error out=w225:errorcluster)
                  n157 = Close Reference(reference=w226, error in (no error)=w225) -> (error out=w215:errorcluster)
                  n158 = call "Temperature vi FGV.vi"("Enum"=Temperature_enum."write", "error in"=w215, "Set Temperature"=0.0, "main ref"=w214) -> ("error out"=→"error out 4":errorcluster)  [unwired: 7 in]
                  n159 = call "HEAVE WRITE FGV.vi"("Enum - Menu"=Heave_Write_enum."WRITE", "error in (no error)"=w215, "main ref"=w214) -> ()  [unwired: 8 in, 1 out]
                }
              }
            }
          }
        }
      }
    }
    frame Error {
    }
  }
  "error out" <- w2
